vi "Initialize.vi"(8 "error in (no error)":errorcluster, 9 "Reset (False)":bool, 11 "VISA resource name":refnum<visa-resource-name>) -> (0 "error out":errorcluster, 3 "VISA resource name out":refnum<visa-resource-name>)   [LabVIEW 2009]
doc: "Establishes communication with the instrument and optionally performs an instrument reset. Therefore, call this VI before calling other instrument driver VIs for this instrument. Generally, you need to call the Initialize VI only once at the beginning of an application."
panel:
  # "(c) 2009 National Instruments.  ALL RIGHTS RESERVED."
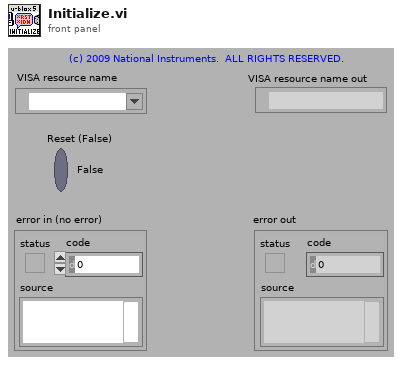
[diagram p1: front panel]
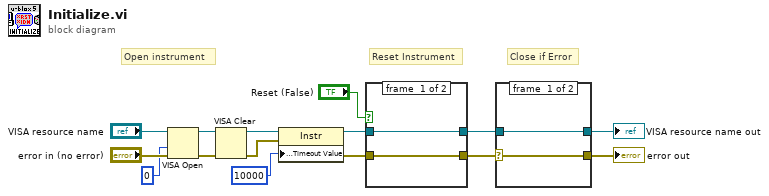
[diagram p0: block diagram]
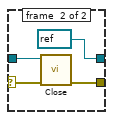
[diagram p2: hidden frame]
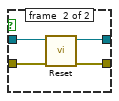
[diagram p3: hidden frame]
diagram:
  # "Close if Error"
  # "Reset Instrument"
  # "Open instrument"
  n1 = VISA Open(access mode=u32 0, error in (no error)="error in (no error)", VISA resource name="VISA resource name") -> (VISA resource name=w10:refnum<visa-resource-name>, error out=w9:errorcluster)  [unwired: 2 out]
  n2 = VISA Clear(VISA resource name=w10, error in (no error)=w9) -> (VISA resource name out=w8:refnum<visa-resource-name>, error out=w7:errorcluster)
  n3 = property class="Instr"(reference=w8, error in=w7, "General Settings:Timeout Value"=u32 10000) -> (reference out=w1:refnum<visa-resource-name>, error out=w2:errorcluster)
  n4 = case shown="True" "Reset (False)" {
    tunnel: w2 -> [w16 w18]
    tunnel: [w16 w21] -> w3
    tunnel: w1 -> [w17 w19]
    tunnel: [w17 w20] -> w4
    frame #0 {
    }
    frame #1 {
      n5 = call "Reset.vi"("error in (no error)"=w18, "VISA resource name"=w19) -> ("error out"=w21:errorcluster, "VISA resource name out"=w20:refnum<visa-resource-name>)  [unwired: 2 in, 6 out]
    }
  }
  n6 = case shown="Error" w3 {
    selector: w3 -> [w22 w25]
    tunnel: w4 -> [w23 w26]
    tunnel: [w23 refnum<visa-resource-name> refnum ("VISA resource name out")] -> w6
    tunnel: [w22 w27] -> w5
    frame #0 {
    }
    frame #1 {
      n7 = call "Close.vi"("error in (no error)"=w25, "VISA resource name"=w26) -> ("error out"=w27:errorcluster)  [unwired: 9 out]
    }
  }
  "VISA resource name out" <- w6
  "error out" <- w5
